vi "Set_AOI_size&position.vi"(6 "error in (no error)":errorcluster, 7 ".NET Refnum in":refnum<k24>, 8 "s32Height":i32, 9 "s32Width":i32, 10 "s32PosY":i32, 11 "s32PosX":i32) -> (0 "error out":errorcluster)   [LabVIEW 2021]
uses:
  C:/Program Files/Thorlabs/Scientific Imaging/ThorCam/uc480DotNet.dll
  Program Files/Thorlabs/Scientific Imaging/ThorCam/uc480DotNet.dll
panel:
  out "Set":i32(ring) items=["SUCCESS, Success"=0, "INVALID_HANDLE"=1, "IO_REQUEST_FAILED"=2, "CANT_OPEN_DEVICE, CaptureStatus"=3, "CANT_CLOSE_DEVICE"=4, "CANT_SETUP_MEMORY"=5, "NO_HWND_FOR_ERROR_REPORT"=6, "ERROR_MESSAGE_NOT_CREATED"=7, "ERROR_STRING_NOT_FOUND"=8, "HOOK_NOT_CREATED"=9, "TIMER_NOT_CREATED"=10, "CANT_OPEN_REGISTRY"=11, "CANT_READ_REGISTRY"=12, "CANT_VALIDATE_BOARD"=13, "CANT_GIVE_BOARD_ACCESS"=14, "NO_IMAGE_MEM_ALLOCATED"=15, "CANT_CLEANUP_MEMORY"=16, "CANT_COMMUNICATE_WITH_DRIVER"=17, "FUNCTION_NOT_SUPPORTED_YET"=18, "OPERATING_SYSTEM_NOT_SUPPORTED"=19, "INVALID_VIDEO_IN"=20, "INVALID_IMG_SIZE"=21, "INVALID_ADDRESS"=22, "INVALID_VIDEO_MODE"=23, "INVALID_AGC_MODE"=24, "INVALID_GAMMA_MODE"=25, "INVALID_SYNC_LEVEL"=26, "INVALID_CBARS_MODE"=27, "INVALID_COLOR_MODE"=28, "INVALID_SCALE_FACTOR"=29, "INVALID_IMAGE_SIZE"=30, "INVALID_IMAGE_POS"=31, "INVALID_CAPTURE_MODE"=32, "INVALID_RISC_PROGRAM"=33, "INVALID_BRIGHTNESS"=34, "INVALID_CONTRAST"=35, "INVALID_SATURATION_U"=36, "INVALID_SATURATION_V"=37, "INVALID_HUE"=38, "INVALID_HOR_FILTER_STEP"=39, "INVALID_VERT_FILTER_STEP"=40, "INVALID_EEPROM_READ_ADDRESS"=41, "INVALID_EEPROM_WRITE_ADDRESS"=42, "INVALID_EEPROM_READ_LENGTH"=43, "INVALID_EEPROM_WRITE_LENGTH"=44, "INVALID_BOARD_INFO_POINTER"=45, "INVALID_DISPLAY_MODE"=46, "INVALID_ERR_REP_MODE"=47, "INVALID_BITS_PIXEL"=48, "INVALID_MEMORY_POINTER"=49, "FILE_WRITE_OPEN_ERROR"=50, "FILE_READ_OPEN_ERROR"=51, "FILE_READ_INVALID_BMP_ID"=52, "FILE_READ_INVALID_BMP_SIZE"=53, "FILE_READ_INVALID_BIT_COUNT"=54, "WRONG_KERNEL_VERSION"=55, "RISC_INVALID_XLENGTH"=60, "RISC_INVALID_YLENGTH"=61, "RISC_EXCEED_IMG_SIZE"=62, "DD_MAIN_FAILED"=70, "DD_PRIMSURFACE_FAILED"=71, "DD_SCRN_SIZE_NOT_SUPPORTED"=72, "DD_CLIPPER_FAILED"=73, "DD_CLIPPER_HWND_FAILED"=74, "DD_CLIPPER_CONNECT_FAILED"=75, "DD_BACKSURFACE_FAILED"=76, "DD_BACKSURFACE_IN_SYSMEM"=77, "DD_MDL_MALLOC_ERR"=78, "DD_MDL_SIZE_ERR"=79, "DD_CLIP_NO_CHANGE"=80, "DD_PRIMMEM_NULL"=81, "DD_BACKMEM_NULL"=82, "DD_BACKOVLMEM_NULL"=83, "DD_OVERLAYSURFACE_FAILED"=84, "DD_OVERLAYSURFACE_IN_SYSMEM"=85, "DD_OVERLAY_NOT_ALLOWED"=86, "DD_OVERLAY_COLKEY_ERR"=87, "DD_OVERLAY_NOT_ENABLED"=88, "DD_GET_DC_ERROR"=89, "DD_DDRAW_DLL_NOT_LOADED"=90, "DD_THREAD_NOT_CREATED"=91, "DD_CANT_GET_CAPS"=92, "DD_NO_OVERLAYSURFACE"=93, "DD_NO_OVERLAYSTRETCH"=94, "DD_CANT_CREATE_OVERLAYSURFACE"=95, "DD_CANT_UPDATE_OVERLAYSURFACE"=96, "DD_INVALID_STRETCH"=97, "EV_INVALID_EVENT_NUMBER"=100, "INVALID_MODE"=101, "CANT_FIND_HOOK, CANT_FIND_FALCHOOK"=102, "CANT_GET_HOOK_PROC_ADDR"=103, "CANT_CHAIN_HOOK_PROC"=104, "CANT_SETUP_WND_PROC"=105, "HWND_NULL"=106, "INVALID_UPDATE_MODE"=107, "NO_ACTIVE_IMG_MEM"=108, "CANT_INIT_EVENT"=109, "FUNC_NOT_AVAIL_IN_OS"=110, "CAMERA_NOT_CONNECTED"=111, "SEQUENCE_LIST_EMPTY"=112, "CANT_ADD_TO_SEQUENCE"=113, "LOW_OF_SEQUENCE_RISC_MEM"=114, "IMGMEM2FREE_USED_IN_SEQ"=115, "IMGMEM_NOT_IN_SEQUENCE_LIST"=116, "SEQUENCE_BUF_ALREADY_LOCKED"=117, "INVALID_DEVICE_ID"=118, "INVALID_BOARD_ID"=119, "ALL_DEVICES_BUSY"=120, "HOOK_BUSY"=121, "TIMED_OUT"=122, "NULL_POINTER"=123, "WRONG_HOOK_VERSION"=124, "INVALID_PARAMETER, InvalidParameter"=125, "NOT_ALLOWED"=126, "OUT_OF_MEMORY"=127, "INVALID_WHILE_LIVE"=128, "ACCESS_VIOLATION"=129, "UNKNOWN_ROP_EFFECT"=130, "INVALID_RENDER_MODE"=131, "INVALID_THREAD_CONTEXT"=132, "NO_HARDWARE_INSTALLED"=133, "INVALID_WATCHDOG_TIME"=134, "INVALID_WATCHDOG_MODE"=135, "INVALID_PASSTHROUGH_IN"=136, "ERROR_SETTING_PASSTHROUGH_IN"=137, "FAILURE_ON_SETTING_WATCHDOG"=138, "NO_USB20"=139, "CAPTURE_RUNNING"=140, "MEMORY_BOARD_ACTIVATED"=141, "MEMORY_BOARD_DEACTIVATED"=142, "NO_MEMORY_BOARD_CONNECTED"=143, "TOO_LESS_MEMORY"=144, "IMAGE_NOT_PRESENT"=145, "MEMORY_MODE_RUNNING"=146, "MEMORYBOARD_DISABLED"=147, "TRIGGER_ACTIVATED"=148, "WRONG_KEY"=150, "CRC_ERROR"=151, "NOT_YET_RELEASED"=152, "NOT_CALIBRATED"=153, "WAITING_FOR_KERNEL"=154, "NOT_SUPPORTED"=155, "TRIGGER_NOT_ACTIVATED"=156, "OPERATION_ABORTED"=157, "BAD_STRUCTURE_SIZE"=158, "INVALID_BUFFER_SIZE"=159, "INVALID_PIXEL_CLOCK"=160, "INVALID_EXPOSURE_TIME"=161, "AUTO_EXPOSURE_RUNNING"=162, "CANNOT_CREATE_BB_SURF"=163, "CANNOT_CREATE_BB_MIX"=164, "BB_OVLMEM_NULL"=165, "CANNOT_CREATE_BB_OVL"=166, "NOT_SUPP_IN_OVL_SURF_MODE"=167, "INVALID_SURFACE"=168, "SURFACE_LOST"=169, "RELEASE_BB_OVL_DC"=170, "BB_TIMER_NOT_CREATED"=171, "BB_OVL_NOT_EN"=172, "ONLY_IN_BB_MODE"=173, "INVALID_COLOR_FORMAT"=174, "INVALID_WB_BINNING_MODE"=175, "INVALID_I2C_DEVICE_ADDRESS"=176, "COULD_NOT_CONVERT"=177, "TRANSFER_ERROR"=178, "PARAMETER_SET_NOT_PRESENT"=179, "INVALID_CAMERA_TYPE"=180, "INVALID_HOST_IP_HIBYTE"=181, "CM_NOT_SUPP_IN_CURR_DISPLAYMODE"=182, "NO_IR_FILTER"=183, "STARTER_FW_UPLOAD_NEEDED"=184, "LIBRARY_NOT_FOUND, DR_LIBRARY_NOT_FOUND"=185, "DR_DEVICE_OUT_OF_MEMORY, DEVICE_OUT_OF_MEMORY"=186, "DR_CANNOT_CREATE_SURFACE, CANNOT_CREATE_SURFACE"=187, "DR_CANNOT_CREATE_VERTEX_BUFFER, CANNOT_CREATE_VERTEX_BUFFER"=188, "CANNOT_CREATE_TEXTURE, DR_CANNOT_CREATE_TEXTURE"=189, "DR_CANNOT_LOCK_OVERLAY_SURFACE, CANNOT_LOCK_OVERLAY_SURFACE"=190, "DR_CANNOT_UNLOCK_OVERLAY_SURFACE, CANNOT_UNLOCK_OVERLAY_SURFACE"=191, "CANNOT_GET_OVERLAY_DC, DR_CANNOT_GET_OVERLAY_DC"=192, "DR_CANNOT_RELEASE_OVERLAY_DC, CANNOT_RELEASE_OVERLAY_DC"=193, "DEVICE_CAPS_INSUFFICIENT, DR_DEVICE_CAPS_INSUFFICIENT"=194, "INCOMPATIBLE_SETTING"=195, "DR_NOT_ALLOWED_WHILE_DC_IS_ACTIVE"=196, "DEVICE_ALREADY_PAIRED"=197, "SUBNETMASK_MISMATCH"=198, "SUBNET_MISMATCH"=199, "INVALID_IP_CONFIGURATION"=200, "DEVICE_NOT_COMPATIBLE"=201, "NETWORK_FRAME_SIZE_INCOMPATIBLE"=202, "NETWORK_CONFIGURATION_INVALID"=203, "ERROR_CPU_IDLE_STATES_CONFIGURATION"=204, "NO_SUCCESS, NoSuccess"=-1]
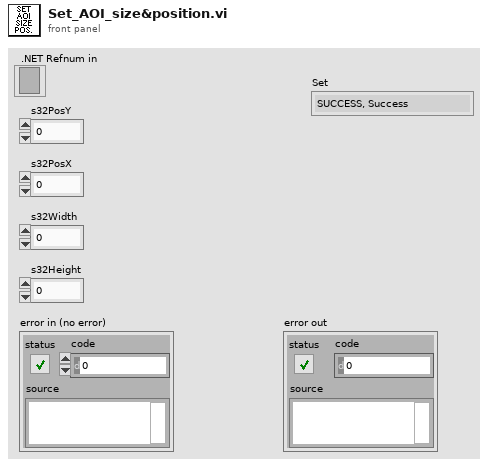
[diagram p1: front panel]
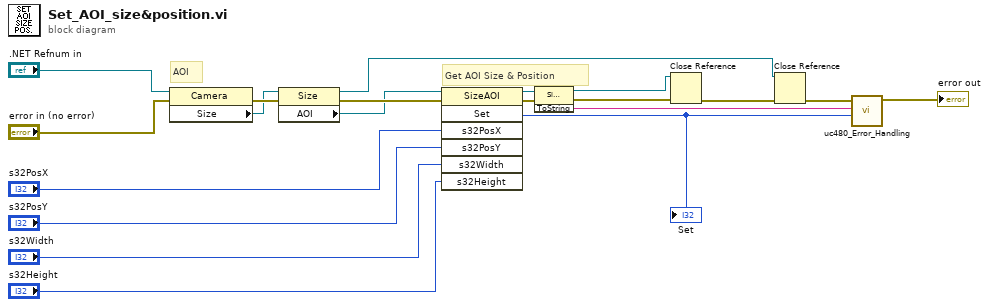
[diagram p0: block diagram]
diagram:
  # "Get AOI Size & Position"
  # "AOI"
  n1 = property class="Camera"(reference=".NET Refnum in", error in="error in (no error)") -> (error out=w6:errorcluster, "Size"=w5:refnum<k24>)  [unwired: 1 out]
  n2 = property class="Size"(reference=w5, error in=w6) -> (reference out=w19:refnum<k24>, error out=w14:errorcluster, "AOI"=w12:refnum<k24>)
  n3 = invoke class="SizeAOI" method="Set"(reference=w12, error in=w14, "s32PosX"="s32PosX", "s32PosY"="s32PosY", "s32Width"="s32Width", "s32Height"="s32Height") -> (reference out=w8:refnum<k24>, error out=w9:errorcluster, "Set"=w10:i32)  [unwired: 1 in, 4 out]
  "Set" <- w10
  n4 = invoke class="SizeAOI" method="ToString"(reference=w8, error in=w9) -> (reference out=w16:refnum<k24>, error out=w15:errorcluster, "ToString"=w7:string)  [unwired: 1 in]
  n5 = Close Reference(reference=w16, error in (no error)=w15) -> (error out=w17:errorcluster)
  n6 = Close Reference(reference=w19, error in (no error)=w17) -> (error out=w18:errorcluster)
  n7 = call "uc480_Error_Handling.vi"("Error Code"=w10, "Error String"=w7, "Error In"=w18) -> ("Error Out"=→"error out":errorcluster)  [unwired: 8 in]
